vi "Read All RAW ADC.vi"(8 "error in (no error)":errorcluster, 10 "# Channels (F:4)":bool, 11 "VISA resource name":refnum<visa-resource-name>) -> (0 "error out":errorcluster, 2 "ADC Raw Values":u16[](array[numeric]) format="%.0x", 3 "VISA resource name out":refnum<visa-resource-name>)   [LabVIEW 2013, in "HadCon.lvlib"]
doc: "Read all ADC raw values, 4 or 8 channels depending on JTAG enabled or disbaled."
uses:
  <instrlib>/HadCon/HadCon.lvlib
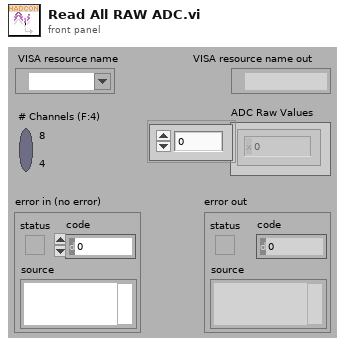
[diagram p1: front panel]
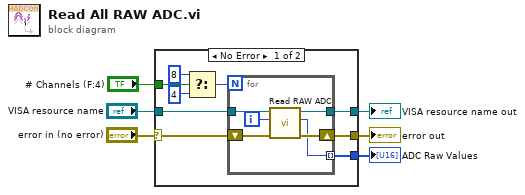
[diagram p0: block diagram]
diagram:
  n1 = case shown="No Error" "error in (no error)" {
    selector: "error in (no error)" -> [w14 w22]
    tunnel: [w12 w23] -> w6
    tunnel: "VISA resource name" -> [w15 w23]
    tunnel: [w13 w22] -> w4
    tunnel: [w11 _] -> w2
    tunnel: "# Channels (F:4)" -> [w10 _]
    frame No Error {
      n2 = Select(t=8, s=w10, f=4) -> (s? t:f=w7:i32)
      n3 = for {
        N: w7 -> [_]
        tunnel: w15 -> [w21]
        tunnel: [w20] -> w12
        shift-right: [w18] -> w13
        shift-left: w14 -> [w19]
        tunnel: [w16] -> w11 mode=indexing
        i -> [w17]
        n4 = call <instrlib>:"Read RAW ADC.vi"("error in (no error)"=w19, "Channel"=w17, "VISA resource name"=w21) -> ("error out"=w18:errorcluster, "ADC Raw Value"=w16:u16, "VISA resource name out"=w20:refnum<visa-resource-name>)  [unwired: 6 in]
      }
    }
    frame Error {
    }
  }
  "VISA resource name out" <- w6
  "error out" <- w4
  "ADC Raw Values" <- w2
